vi "Main.vi"() -> ()   [LabVIEW 2016]
doc: "\"Discrete LED demo.vi\" -- Demonstrate a discrete LED connected to a digital output.\n\nInstructions:\n\n-- Click the 'enable blinker' button to toggle between blinking mode\nand static mode.\n-- In static mode, click the 'digital level' button to set the state of the\ndigital output.\n-- The 'digital output state' LED indicator shows the state of the\ndigital output (on = high, off = low)."
uses:
  <vilib>/vision/Image Controls.llb/IMAQ Image.ctl
  <vilib>/myRIO/Instrument Drivers/Onboard IO/PWM/typedefs/PWM Reference.ctl
  <vilib>/myRIO/Common/Instrument Driver Framework/Utilities/typedefs/myRIO Generic Hardware Reference.ctl
  <vilib>/myRIO/Common/Instrument Driver Framework/Utilities/typedefs/Hardware Version Enum.ctl
  <vilib>/myRIO/Common/Instrument Driver Framework/Utilities/typedefs/myRIO v1.0 Reference.ctl
  <vilib>/myRIO/Common/Instrument Driver Framework/Utilities/typedefs/Generic FPGA Reference.ctl
  <vilib>/myRIO/Common/Instrument Driver Framework/myRIO v1.0/PWM/typedefs/PWM Channels Enum.ctl
  <vilib>/myRIO/Instrument Drivers/Onboard IO/PWM/typedefs/PWM Configuration.ctl
  <vilib>/userdefined/High Color/nirio_resource_hc.ctl
  <vilib>/myRIO/Instrument Drivers/Onboard IO/DIO/typedefs/DIO Reference.ctl
  <vilib>/myRIO/Common/Instrument Driver Framework/myRIO v1.0/DIO/typedefs/DIO Channels List.ctl
  <vilib>/myRIO/Common/Instrument Driver Framework/myRIO v1.0/DIO/typedefs/DIO Channels Enum.ctl
  <vilib>/myRIO/Common/Instrument Driver Framework/myRIO v1.0/Encoder/typedefs/Encoder Signal Mode.ctl
  <vilib>/myRIO/Instrument Drivers/Onboard IO/Encoder/typedefs/Encoder Reference.ctl
  <vilib>/myRIO/Common/Instrument Driver Framework/myRIO v1.0/Encoder/typedefs/Encoder Channels Enum.ctl
  <vilib>/myRIO/Common/Instrument Driver Framework/myRIO v1.0/Encoder/typedefs/Encoder Configuration v1.0.ctl
  <vilib>/myRIO/Common/Instrument Driver Framework/Utilities/vis/Is FPGA Ref Available.vi
  <vilib>/myRIO/Common/Instrument Driver Framework/myRIO v1.0/PWM/vis/myRIO v1.1 Open PWM.vi
  <vilib>/myRIO/Common/Instrument Driver Framework/myRIO v1.0/DIO/vis/myRIO v1.1 Open DIO.vi
  <vilib>/myRIO/Instrument Drivers/Onboard IO/DIO/vis/Write.vi
  <vilib>/myRIO/Common/Instrument Driver Framework/myRIO v1.0/Encoder/vis/myRIO v1.1 Open Encoder.vi
  <vilib>/myRIO/Instrument Drivers/Onboard IO/Encoder/vis/Read.vi
  <vilib>/myRIO/Common/Instrument Driver Framework/Utilities/vis/Validate Channels.vi
  <vilib>/myRIO/Common/Instrument Driver Framework/myRIO v1.0/PWM/vis/myRIO v1.0 Reserve PWM.vi
  <vilib>/myRIO/Common/Instrument Driver Framework/myRIO v1.0/DIO/vis/myRIO v1.0 Reserve DIO.vi
  <vilib>/myRIO/Common/Instrument Driver Framework/myRIO v1.0/Encoder/vis/myRIO v1.0 Reserve Encoder.vi
  <vilib>/myRIO/Common/Instrument Driver Framework/myRIO v1.0/UART/vis/myRIO v1.0 Close UART.vi
  <vilib>/myRIO/Common/Instrument Driver Framework/myRIO v1.0/PWM/vis/myRIO v1.0 Build MUX Configuration PWM.vi
  <vilib>/myRIO/Common/Instrument Driver Framework/myRIO v1.0/Resource Manager/vis/myRIO v1.0 Reserve Channel List.vi
  <vilib>/myRIO/Common/Instrument Driver Framework/myRIO v1.0/DIO/vis/myRIO v1.0 Build MUX Configuration DIO.vi
  <vilib>/myRIO/Common/Instrument Driver Framework/myRIO v1.0/Encoder/vis/myRIO v1.0 Build MUX Configuration Encoder.vi
  <vilib>/myRIO/Common/Instrument Driver Framework/myRIO v1.0/Resource Manager/vis/myRIO v1.0 Create Configuration List.vi
  <vilib>/myRIO/Common/Instrument Driver Framework/myRIO v1.0/Resource Manager/vis/myRIO v1.0 Reserve Channel.vi
  <vilib>/myRIO/Common/Instrument Driver Framework/myRIO v1.0/Resource Manager/vis/myRIO v1.0 Unreserve Channel.vi
  <vilib>/myRIO/Common/Instrument Driver Framework/myRIO v1.0/Resource Manager/vis/myRIO v1.0 Build Mutex Name.vi
  <vilib>/Utility/VariantDataType/GetNumericInfo.vi
  <vilib>/Utility/error.llb/Error Cluster From Error Code.vi
  <vilib>/myRIO/Common/Instrument Driver Framework/myRIO v1.0/myRIO v1.1 Open.vi
  <vilib>/myRIO/Common/Instrument Driver Framework/Utilities/vis/IO Manager.vi
  <vilib>/myRIO/Common/Instrument Driver Framework/Utilities/vis/Configuration Manager.vi
  <vilib>/myRIO/Common/Instrument Driver Framework/myRIO v1.0/Resource Manager/vis/myRIO v1.0 Configure IO.vi
  <vilib>/myRIO/Common/Instrument Driver Framework/myRIO v1.0/myRIO v1.0 Close.vi
  <vilib>/myRIO/Common/Instrument Driver Framework/myRIO v1.0/PWM/vis/myRIO v1.0 Write PWM.vi
  <vilib>/myRIO/Common/Instrument Driver Framework/myRIO v1.0/DIO/vis/myRIO v1.0 Write DIO.vi
  <vilib>/myRIO/Common/Instrument Driver Framework/myRIO v1.0/Encoder/vis/myRIO v1.0 Configure Encoder.vi
  <vilib>/myRIO/Common/Instrument Driver Framework/myRIO v1.0/Encoder/vis/myRIO v1.0 Read Encoder.vi
  <vilib>/myRIO/Common/Instrument Driver Framework/Utilities/vis/FPGA Ref Manager.vi
  <vilib>/myRIO/Common/Instrument Driver Framework/myRIO v1.0/myRIO v1.0 Reset FPGA.vi
  <vilib>/myRIO/Common/Instrument Driver Framework/myRIO v1.0/IRQ/vis/myRIO v1.0 IRQ Info FGV.vi
  <vilib>/myRIO/Common/Instrument Driver Framework/myRIO v1.0/IRQ/vis/myRIO v1.0 Timer IRQ Info FGV.vi
  <vilib>/myRIO/Common/Instrument Driver Framework/myRIO v1.0/IRQ/vis/myRIO v1.0 ISR Agent.vi
  <vilib>/myRIO/Express VI/Onboard IO/PWM/PWM Express VI.xnode
  <vilib>/myRIO/Instrument Drivers/Onboard IO/PWM/vis/myRIO PWM Open.xnode
  <vilib>/myRIO/Express VI/Onboard IO/DO/DO Express VI.xnode
  <vilib>/myRIO/Instrument Drivers/Onboard IO/DIO/vis/myRIO DIO Open.xnode
  <vilib>/myRIO/Express VI/Onboard IO/Encoder/Encoder Express VI.xnode
  <vilib>/myRIO/Instrument Drivers/Onboard IO/Encoder/vis/myRIO Encoder Open.xnode
  <vilib>/myRIO/Common/Instrument Driver Framework/myRIO v1.0/Encoder/typedefs/Encoder Count Direction Enum.ctl
  <vilib>/myRIO/Instrument Drivers/Utilities/Utilities.lvlib
  <vilib>/myRIO/Instrument Drivers/Onboard IO/PWM/PWM.lvlib
  <vilib>/myRIO/Instrument Drivers/Onboard IO/DIO/DIO.lvlib
  <vilib>/myRIO/Instrument Drivers/Onboard IO/Encoder/Encoder.lvlib
panel:
  out "All Image Buffers Out":T1[](array[typedef])
  out "offset [%FS]":dbl
  in  "null offset":bool
  out "duty cycle [%]":dbl
  out "pulse width [ms]":dbl=1.5
  in  "freq [Hz]":dbl=50.0
  in  "position [%FS]":dbl(slide) scale=-200.0..200.0
  out "CamStopped":bool caption="Stopped"
  in  "StopCam (F)":bool caption="Stop (F)"
  out "Image Out":T1(plugin-control)
  out "Counter Value":i32
  out "Boolean 2":bool
  out "back":bool
  out "Reset Counter":bool
  in  "PWM 2":dbl(slide)=0.5 scale=0.0..1.0
  in  "PWM 1":dbl(slide)=0.5 scale=0.0..1.0
  in  "Stop Button":bool
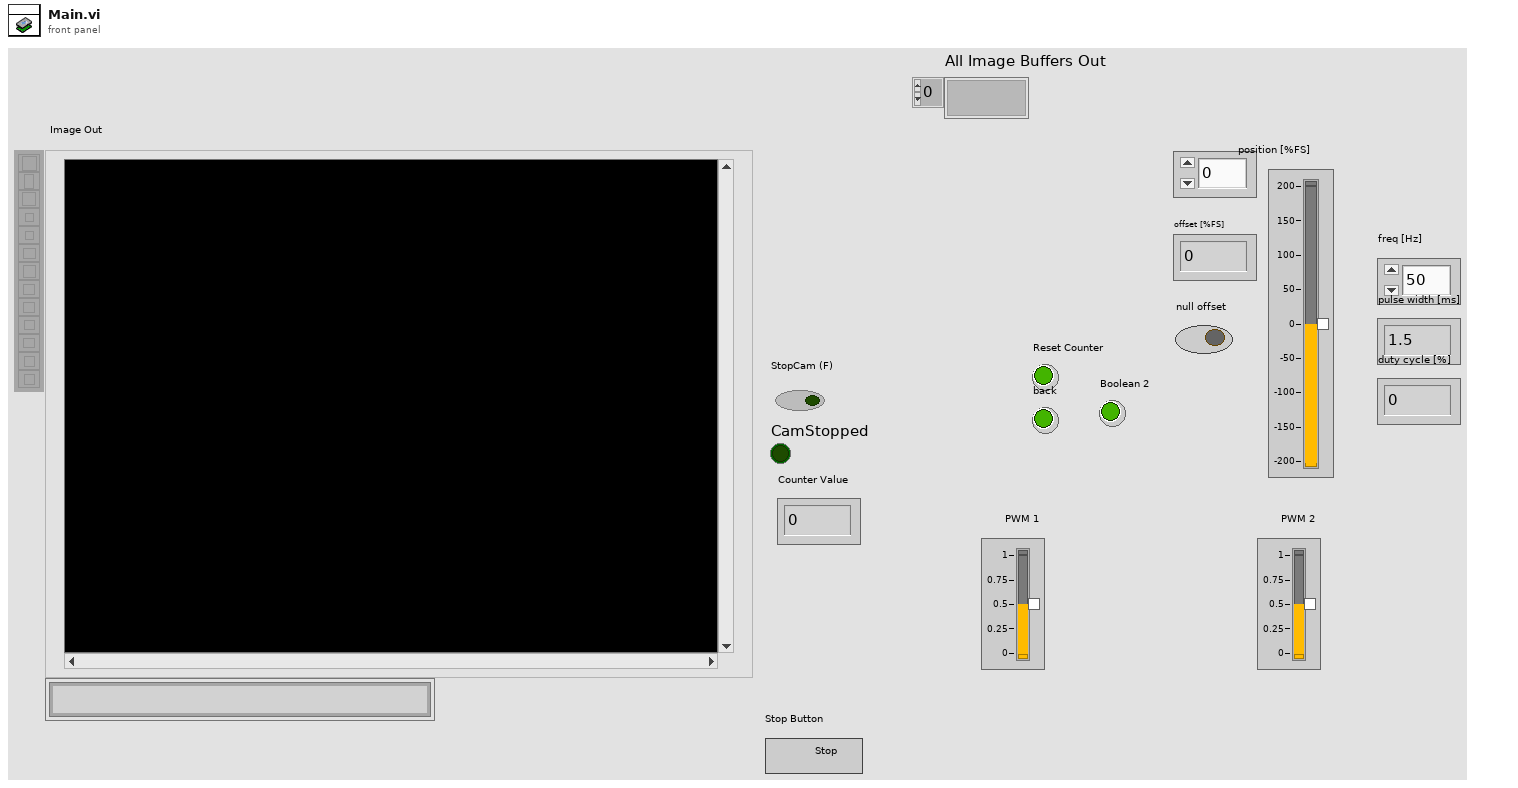
[diagram p1: front panel]
types:
  T1 = typedef "IMAQ Image.ctl" = refnum<image>
  T2 = typedef "PWM.lvlib/PWM Reference.ctl" = cluster{"myRIO Reference":T3, "PWM Channels Enum":T7, "PWM Configuration":T8}
  T3 = typedef "myRIO Generic Hardware Reference.ctl" = cluster{"myRIO Model":T4, "myRIO Hardware Reference":T5}
  T4 = typedef "Hardware Version Enum.ctl" = enum16{"Unknown", "myRIO-1900", "myRIO-1950", "roboRIO", "NI ELVIS RIO CM"}
  T5 = typedef "myRIO v1.0 Reference.ctl" = cluster{"Generic FPGA Reference":T6, "Allow multiple opens":bool}
  T6 = typedef "Generic FPGA Reference.ctl" = refnum<k20>
  T7 = typedef "PWM Channels Enum.ctl" = enum16{"Not Connected", "C/PWM0", "C/PWM1", "A/PWM0", "A/PWM1", "A/PWM2", "B/PWM0", "B/PWM1", "B/PWM2", "PWM/PWM0", "PWM/PWM1", "PWM/PWM2", "PWM/PWM3", "PWM/PWM4", "PWM/PWM5", "PWM/PWM6", "PWM/PWM7", "PWM/PWM8", "PWM/PWM9"}
  T8 = typedef "PWM.lvlib/PWM Configuration.ctl" = cluster{"Frequency":dbl, "Duty Cycle":dbl}
  T9 = typedef "nirio_resource_hc.ctl" = tag
  T10 = typedef "Encoder.lvlib/Encoder Reference.ctl" = cluster{"myRIO Reference":T3, "Encoder Channels Enum":T11}
  T11 = typedef "Encoder Channels Enum.ctl" = enum16{"Not Connected", "C/ENC0", "C/ENC1", "A/ENC", "B/ENC", "DIO/ENC0", "DIO/ENC1", "DIO/ENC2", "DIO/ENC3", "DIO/ENC4"}
  T12 = typedef "Encoder Signal Mode.ctl" = enum16{"Quadrature phase signal", "Step and direction signal"}
  T13 = typedef "DIO.lvlib/DIO Reference.ctl" = cluster{"myRIO Reference":T3, "DIO Channels List":T14}
  T14 = typedef "DIO Channels List.ctl" = T15[]
  T15 = typedef "DIO Channels Enum.ctl" = enum16{"Not Connected", "C/DIO0", "C/DIO1", "C/DIO2", "C/DIO3", "C/DIO4", "C/DIO5", "C/DIO6", "C/DIO7", "A/DIO0", "A/DIO1", "A/DIO2", "A/DIO3", "A/DIO4", "A/DIO5", "A/DIO6", "A/DIO7", "A/DIO8", "A/DIO9", "A/DIO10", "A/DIO11", "A/DIO12", "A/DIO13", "A/DIO14", "A/DIO15", "B/DIO0", "B/DIO1", "B/DIO2", "B/DIO3", "B/DIO4", "B/DIO5", "B/DIO6", "B/DIO7", "B/DIO8", "B/DIO9", "B/DIO10", "B/DIO11", "B/DIO12", "B/DIO13", "B/DIO14", "B/DIO15", "LED0", "LED1", "LED2", "LED3", "Button0", "DIO/DIO0", "DIO/DIO1", "DIO/DIO2", "DIO/DIO3", "DIO/DIO4", "DIO/DIO5", "DIO/DIO6", "DIO/DIO7", "DIO/DIO8", "DIO/DIO9", "SPI/CS0", "SPI/CS1", "SPI/CS2", "SPI/CS3", "LED RADIO (Green)", "LED RADIO (Red)", "LED COMM (Green)", "LED COMM (Red)", "LED MODE (Green)", "LED MODE (Red)"}
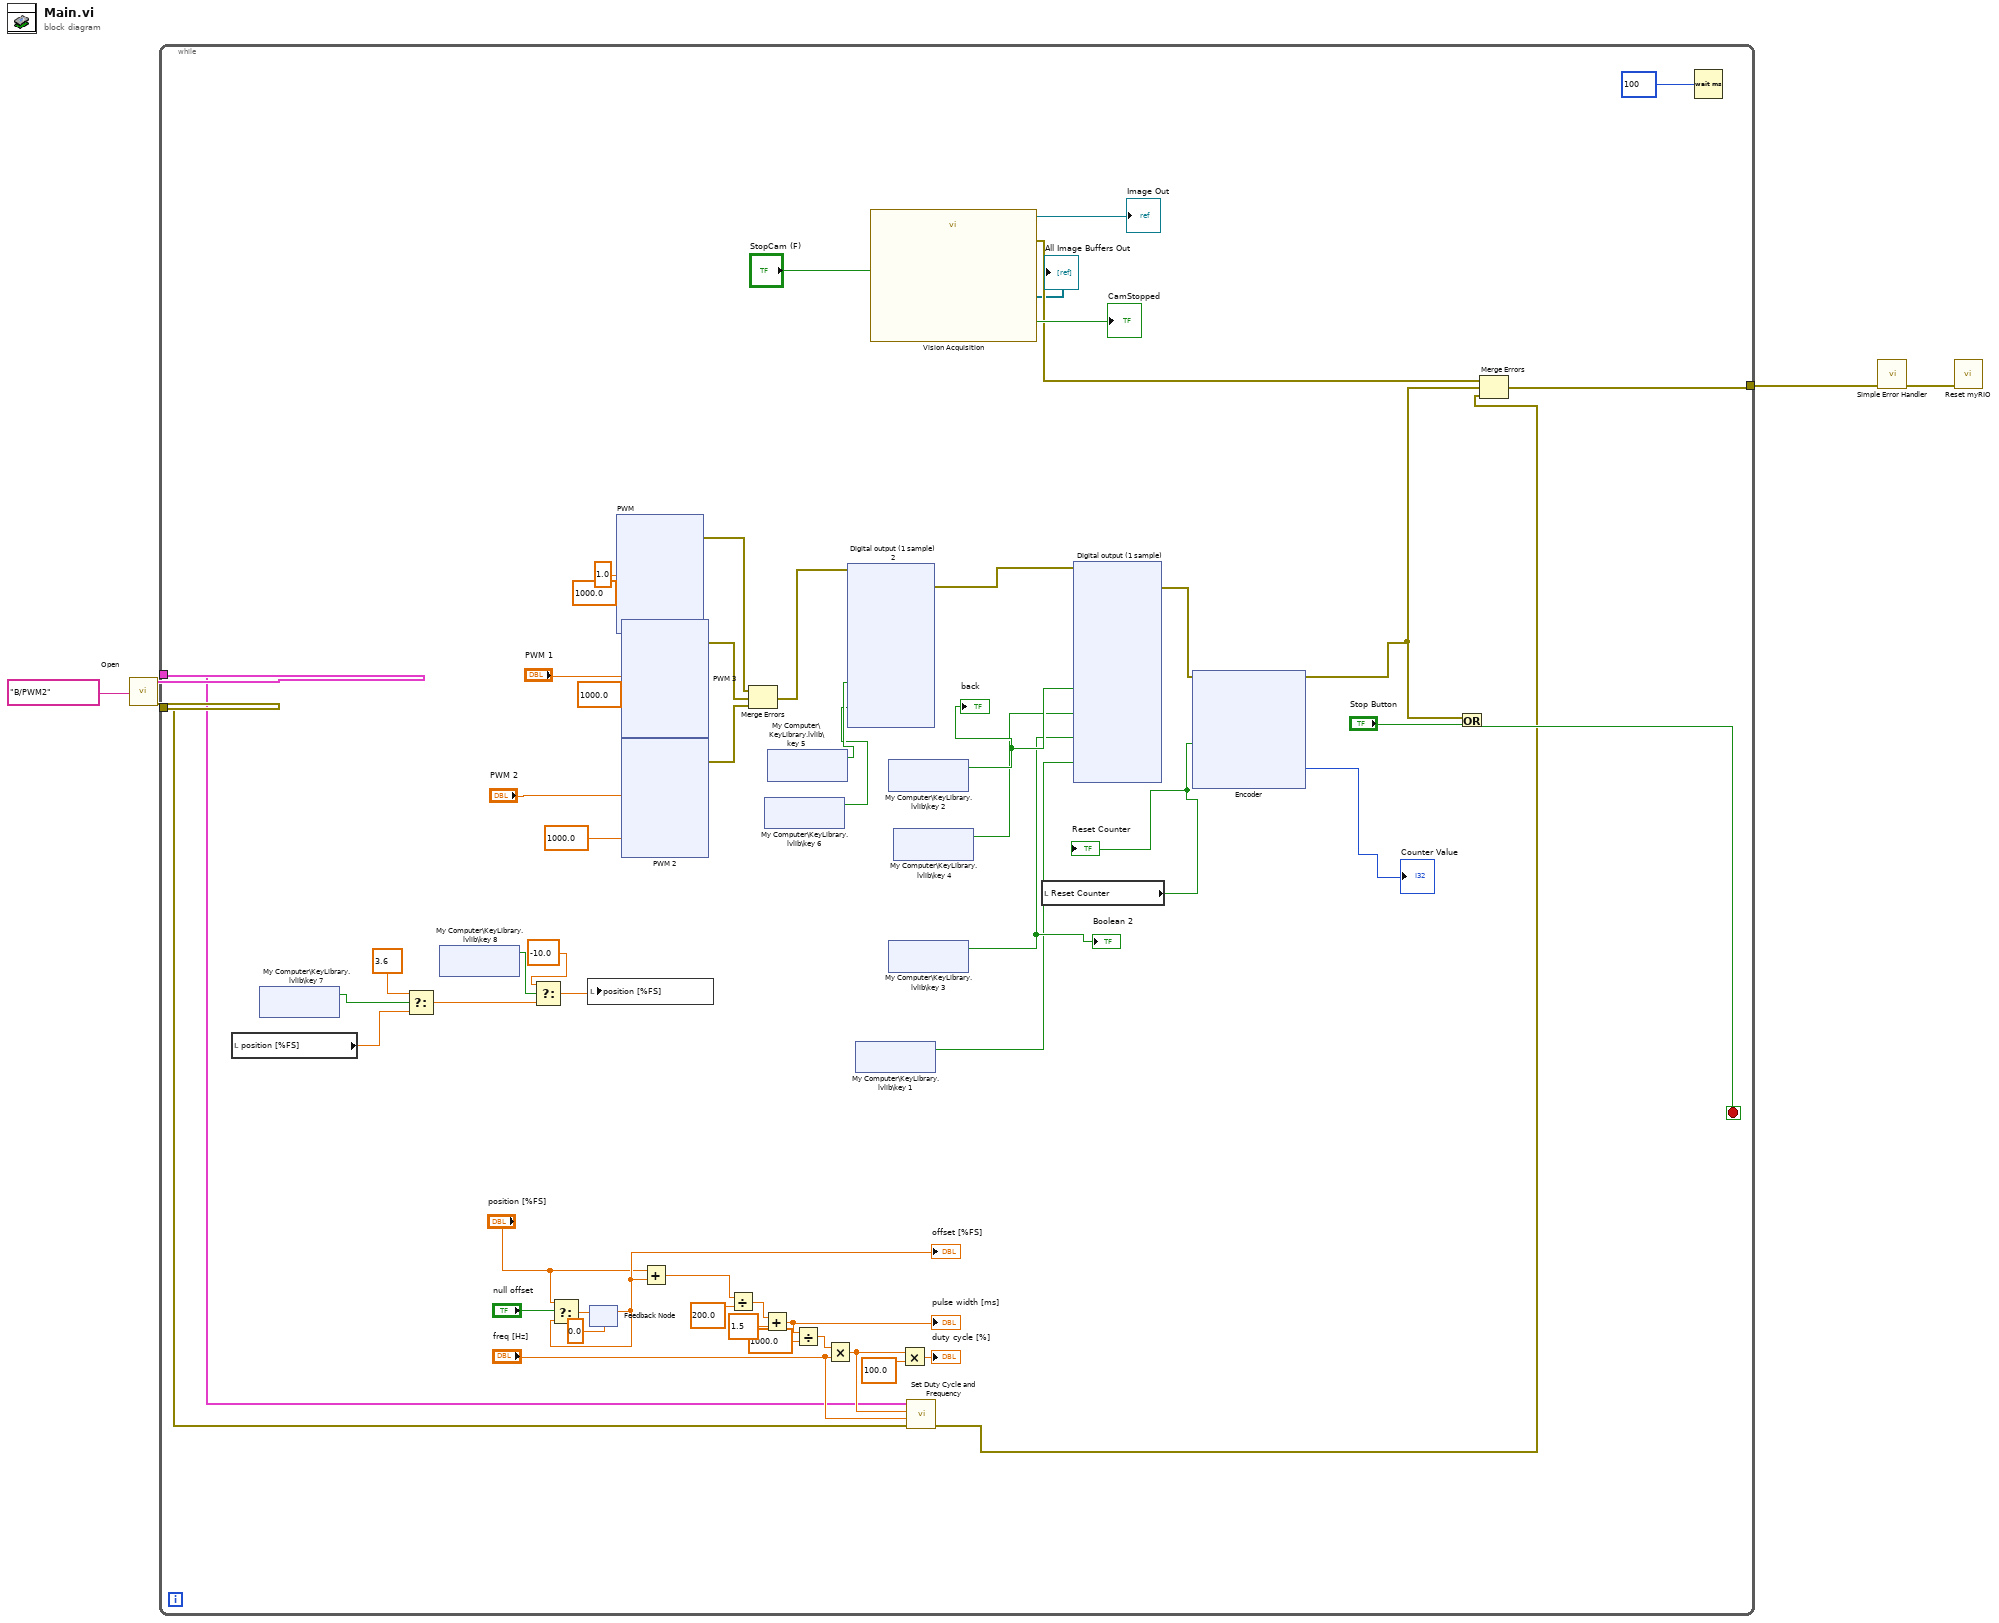
[diagram p0: block diagram]
diagram:
  n1 = call <vilib>:"Open.vi"("Channel Name"=tag "B/PWM2" ("PWM channel")) -> ("error out"=w3:errorcluster, "PWM Ref Out"=w2:T2)  [unwired: 9 in]
  n2 = while {
    tunnel: [w40] -> w1
    tunnel: w3 -> [w16]
    tunnel: w2 -> [w17]
    stop <- w60 stop-if-true
    n3 = local read "position [%FS]"() -> (w7:dbl)
    n4 = shared-variable "My Computer\\KeyLibrary.lvlib\\key 7"() -> (w13:bool)  [unwired: 1 in, 1 out]
    n5 = Select(t=3.6 ("x"), s=w13, f=w7) -> (s? t:f=w11:dbl)
    n6 = shared-variable "My Computer\\KeyLibrary.lvlib\\key 8"() -> (w10:bool)  [unwired: 1 in, 1 out]
    n7 = Select(t=-10.0 ("x"), s=w10, f=w11) -> (s? t:f=w8:dbl)
    n8 = local write "position [%FS]"(w8) -> ()
    n9 = feedback #1(0.0 ("position [%FS]")) -> (w24:dbl)
    "offset [%FS]" <- w24
    n10 = Select(t="position [%FS]", s="null offset", f=w24) -> (s? t:f=w26:dbl)
    n11 = feedback-in #1(w26) -> ()
    n12 = xnode "PWM"("Duty Cycle"=1.0, "Frequency [Hz]"=1000.0) -> ("error out"=w49:errorcluster)  [unwired: 1 in]
    n13 = xnode "PWM 3"("Duty Cycle"="PWM 1", "Frequency [Hz]"=1000.0) -> ("error out"=w59:errorcluster)  [unwired: 1 in]
    n14 = xnode "PWM 2"("Duty Cycle"="PWM 2", "Frequency [Hz]"=1000.0) -> ("error out"=w58:errorcluster)  [unwired: 1 in]
    n15 = Add(x="position [%FS]", y=w24) -> (x+y=w25:dbl)
    n16 = Divide(x=w25, y=200.0) -> (x/y=w32:dbl)
    n17 = Merge Errors(w49, w59, w58) -> (w53:errorcluster)
    n18 = Add(x=w32, y=1.5) -> (x+y=w30:dbl)
    "pulse width [ms]" <- w30
    n19 = shared-variable "My Computer\\KeyLibrary.lvlib\\key 6"() -> (w34:bool)  [unwired: 1 in, 1 out]
    n20 = shared-variable "My Computer\\KeyLibrary.lvlib\\key 5"() -> (w35:bool)  [unwired: 1 in, 1 out]
    n21 = Divide(x=w30, y=1000.0) -> (x/y=w22:dbl)
    n22 = Multiply(x=w22, y="freq [Hz]") -> (x*y=w19:dbl)
    n23 = xnode "Digital output (1 sample) 2"("B/DIO5 (Pin 21)"=w35, "B/DIO6 (Pin 23)"=w34, "error in (no error)"=w53) -> ("error out"=w46:errorcluster)
    n24 = shared-variable "My Computer\\KeyLibrary.lvlib\\key 1"() -> (w42:bool)  [unwired: 1 in, 1 out]
    n25 = call "Vision Acquisition"("Stop (F)"="StopCam (F)") -> ("Image Out"=→"Image Out":T1, "All Image Buffers Out"=→"All Image Buffers Out":T1[], "Stopped"=→"CamStopped":bool, "error out"=w36:errorcluster)  [unwired: 23 in]
    n26 = shared-variable "My Computer\\KeyLibrary.lvlib\\key 2"() -> (w45:bool)  [unwired: 1 in, 1 out]
    "back" <- w45
    n27 = shared-variable "My Computer\\KeyLibrary.lvlib\\key 3"() -> (w44:bool)  [unwired: 1 in, 1 out]
    "Boolean 2" <- w44
    n28 = shared-variable "My Computer\\KeyLibrary.lvlib\\key 4"() -> (w43:bool)  [unwired: 1 in, 1 out]
    n29 = Multiply(x=w19, y=100.0) -> (x*y=→"duty cycle [%]":dbl)
    n30 = call <vilib>:"Set Duty Cycle and Frequency.vi"("error in (no error)"=w16, "Frequency [Hz]"="freq [Hz]", "Duty Cycle"=w19, "PWM Ref In"=w17) -> ("error out"=w15:errorcluster)  [unwired: 5 in, 1 out]
    n31 = local read "Reset Counter"() -> (w50:bool)
    "Reset Counter" <- w50
    n32 = xnode "Digital output (1 sample)"("A/DIO5 (Pin 21)"=w45, "A/DIO6 (Pin 23)"=w43, "A/DIO7 (Pin 25)"=w44, "A/DIO13 (Pin 26)"=w42, "error in (no error)"=w46) -> ("error out"=w52:errorcluster)
    n33 = xnode "Encoder"("Reset Counter"=w50, "error in (no error)"=w52) -> ("Counter Value"=→"Counter Value":i32, "error out"=w41:errorcluster)  [unwired: 2 out]
    n34 = Or(x=w41, y="Stop Button") -> (x .or. y?=w60:bool)
    n35 = Merge Errors(w36, w41, w15) -> (w40:errorcluster)
    n36 = Wait (ms)(milliseconds to wait=u32 100 ("millisecond timer value")) -> ()  [unwired: 1 out]
  }
  n37 = call <vilib>:"Simple Error Handler.vi"("error in (no error)"=w1) -> ("error out"=w5:errorcluster)  [unwired: 4 in, 4 out]
  n38 = call <vilib>:"Reset myRIO.vi"("error in (no error)"=w5) -> ()  [unwired: 10 in, 1 out]
